vi "Reset Keithley over Time.vi"(6 "Reset Button":bool, 7 "Data":dbl[][](array[numeric]), 8 "Time Stamp Iteration":timestamp, 9 "Time Array IN":dbl[](array[numeric]), 10 "Iteration Number":i32, 11 "Mean and SD":dbl[][](array[numeric])) -> (0 "Time Stamp Iteration out":timestamp, 1 "Time Array OUT":dbl[](array[numeric]), 2 "Iteration Number out":i32, 3 "Mean and SD out":dbl[][](array[numeric]), 5 "Data out":dbl[][](array[numeric]))   [LabVIEW 2018]
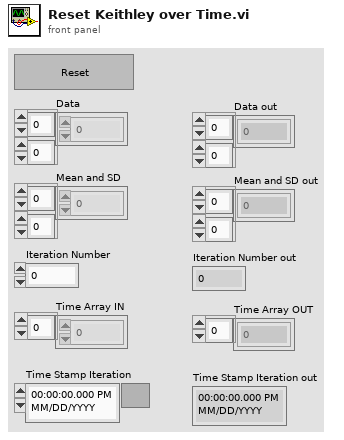
[diagram p1: front panel]
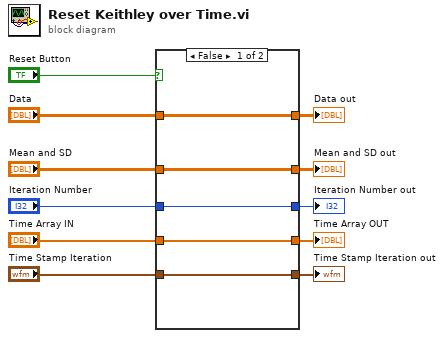
[diagram p0: block diagram]
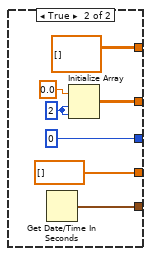
[diagram p2: hidden frame]
diagram:
  n1 = case shown="False" "Reset Button" {
    tunnel: [w16 dbl[][] []] -> w5
    tunnel: [w15 w20] -> w4
    tunnel: [w13 dbl[] [] ("Time Array OUT")] -> w2
    tunnel: [w12 w18] -> w1
    tunnel: [w14 0] -> w3
    tunnel: "Data" -> [w16 _]
    tunnel: "Mean and SD" -> [w15 _]
    tunnel: "Iteration Number" -> [w14 _]
    tunnel: "Time Array IN" -> [w13 _]
    tunnel: "Time Stamp Iteration" -> [w12 _]
    frame False {
    }
    frame True {
      w22 = 2 ("dimension size")
      n2 = Get Date/Time In Seconds() -> (seconds since 1Jan1904=w18:timestamp)
      n3 = Initialize Array(0.0 ("element"), w22, w22) -> (w20:dbl[][])
    }
  }
  "Data out" <- w5
  "Mean and SD out" <- w4
  "Iteration Number out" <- w3
  "Time Array OUT" <- w2
  "Time Stamp Iteration out" <- w1
